vi "setUp.vi"(8 "error in (no error)":errorcluster, 11 "reference in":refnum<class "DSF CD GE Reflective Memory System Tests.lvclass">=refnum) -> (0 "error out":errorcluster, 3 "reference out":refnum<class "DSF CD GE Reflective Memory System Tests.lvclass">)   [LabVIEW 2021, in "DSF CD GE Reflective Memory System Tests.lvclass"]
doc: "setUp runs prior to the test method during test execution. Use this method to initialize any object data required by your tests."
uses:
  DSF CD GE Reflective Memory System Tests.lvclass
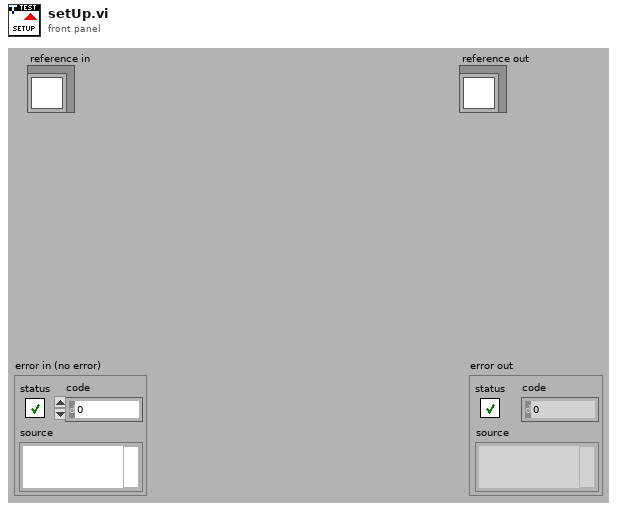
[diagram p1: front panel]
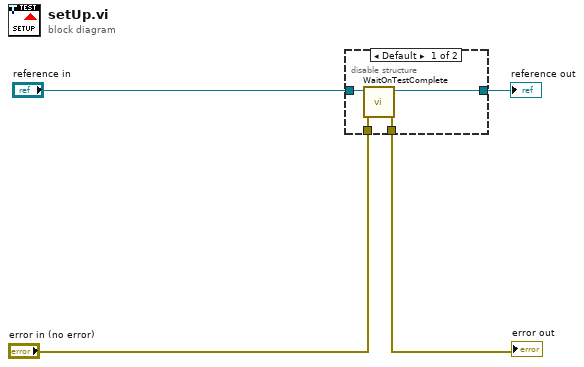
[diagram p0: block diagram]
diagram:
  n1 = disable-structure shown="Default" {
    disable-tunnel: "error in (no error)" -> [w8 w9]
    disable-tunnel: [w7 w9] -> w4
    disable-tunnel: [w6 w10] -> w3
    disable-tunnel: "reference in" -> [w5 w10]
    frame condition #0 (active) {
      n2 = call <vilib>:"WaitOnTestComplete.vi"("error in (no error)"=w8, "TestCase in"=w5) -> ("error out"=w7:errorcluster, "TestCase out"=w6:refnum<class "DSF CD GE Reflective Memory System Tests.lvclass">)  [unwired: 8 in]
    }
    frame condition #1 {
    }
  }
  "error out" <- w4
  "reference out" <- w3
